vi "Subvi galvo 1.vi"(8 "Ext trig enable":bool, 10 "FIFO In":refnum<k21>="AB0") -> ()   [LabVIEW 2017]
uses:
  <vilib>/rvi/Emulation/niFpgaGetClockAttributes.vi
  <vilib>/rvi/Emulation/niFpgaSctlEmulationGetInTimedLoop.vi
  <vilib>/rvi/Emulation/niFpgaEmulationReportErrorSimple.vi
  GV FIFO timeout.vi
  <vilib>/rvi/eio/common/nirviEmuTemplateMethod_errors.vi
  <vilib>/rvi/DataTransferAndStorage/Container/Common/niFpgaContainerExecOnDevCompGetState.vi
  <vilib>/rvi/Emulation/niFpgaEmulationIsFPGAContextNoSignature.vi
  <vilib>/rvi/errors/niFpgaSetErrorForExecOnDevCompSimple.vi
  <vilib>/rvi/eio/common/nirviEmuReportErrorAndStop.vi
  <vilib>/rvi/DataTransferAndStorage/Container/Common/niFpgaContainerGetUniqueNameForEmu.vi
  <vilib>/rvi/FIFO/Fifo_Resource/nirvififoEmulationSetSize.vi
  <vilib>/rvi/FIFO/Fifo_Resource/nirviFifoEmulationQueueMgr.vi
  <instcachedir>/0/nirviFifoEmulationQueueMgr_E5CAEC123FF24DC58D834DCA3CDAA9B5.lvgen/nirviFifoEmulationQueueMgr_E5CAEC123FF24DC58D834DCA3CDAA9B5_001.vi
  <vilib>/rvi/FIFO/Fifo_Resource/nirvififoEmulationDetermineInputValidOut.vi
  <vilib>/rvi/FIFO/Fifo_Resource/nirvififoEmulationCreateLock.vi
  <vilib>/rvi/Emulation/niFpgaProcessEmulError.vi
  <vilib>/rvi/FIFO/Fifo_Resource/nirvififoEmulationObtainLock.vi
  <vilib>/rvi/FIFO/Fifo_Resource/nirvififoEmulationReleaseLock.vi
  <vilib>/rvi/occurrence/nirviWaitOnOccurrenceBase.vi
  <vilib>/rvi/errors/nirviReportUnexpectedCaseInternalError.vi
  <vilib>/rvi/errors/nirviReportUnexpectedCaseInternalError (U32).vi
  <vilib>/Utility/error.llb/Clear Errors.vi
  <vilib>/rvi/interface/RandomDataEmulation/niFpgaRandomDataHandleErrors.vi
  <vilib>/rvi/Emulation/niFpgaCriticalErrorInLSC.vi
  <vilib>/eio/EIONode/EIONode.xnode
  <vilib>/rvi/DataTransferAndStorage/Container/XNode/niFpgaContainer.xnode
  <vilib>/rvi/FIFO/Fifo_Resource/niFpgaFifoEmulationRefIn.vi
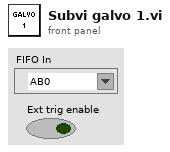
[diagram p1: front panel]
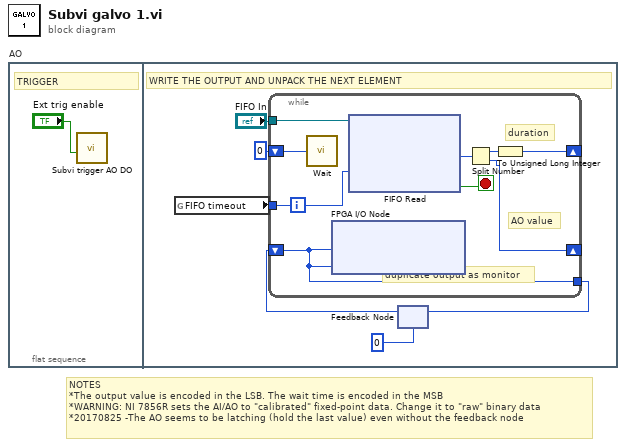
[diagram p0: block diagram]
diagram:
  # "NOTES\n*The output value is encoded in the LSB. The wait time is encoded in the MSB\n*WARNING: NI 7856R sets the AI/AO to \"calibrated\" fixed-point data. Change it to \"raw\" binary data\n*20170825 -The AO seems to be latching (hold the last value) even without the feedback node"
  n1 = flat-sequence "AO" {
    frame #0 {
      # "TRIGGER"
      n2 = call "Subvi trigger AO DO.vi"("Ext trig enable"="Ext trig enable") -> ()  [unwired: 11 in]
    }
    frame #1 {
      # "WRITE THE OUTPUT AND UNPACK THE NEXT ELEMENT"
      n3 = global read "GV FIFO timeout.vi" "FIFO timeout"() -> (w3:i32)
      n4 = feedback #1(u16 0) -> (w6:u16)
      n5 = while {
        shift-right: [w9] -> _
        shift-left: u32 0 -> [w16]
        shift-right: [w14] -> _
        shift-left: w6 -> [w8]
        tunnel: [w8] -> w4
        tunnel: "FIFO In" -> [w11]
        tunnel: w3 -> [w10]
        stop <- w12 stop-if-true
        # "duplicate output as monitor"
        # "duration"
        # "AO value"
        n6 = call "Wait"("Count(Ticks)"=w16) -> ()  [unwired: 1 out]
        n7 = xnode "FPGA I/O Node"("Connector1/AO0"=w8, "Connector1/AO1"=w8) -> ()  [unwired: 2 in, 2 out]
        n8 = xnode ("FIFO Read")("Timeout"=w10, "FIFO In"=w11) -> ("Element"=w13:u32, "Timed Out?"=w12:bool)  [unwired: 1 out]
        n9 = Split Number(x=w13) -> (hi(x)=w15:u16, lo(x)=w14:u16)
        n10 = To Unsigned Long Integer(number=w15) -> (unsigned 32bit integer=w9:u32)
      }
      n11 = feedback-in #1(w4) -> ()
    }
  }
